vi "CodifyFrequency(Array).vi"(1 "Array":dbl[](array[numeric]) min=60.0 max=90.0 step=0.1) -> (0 "Array 2":u32[](array[numeric]))   [LabVIEW 2017, in "AODControl.lvlib"]
uses:
  AODControl.lvlib
panel:
  out "Boolean array":bool[](array[boolean])
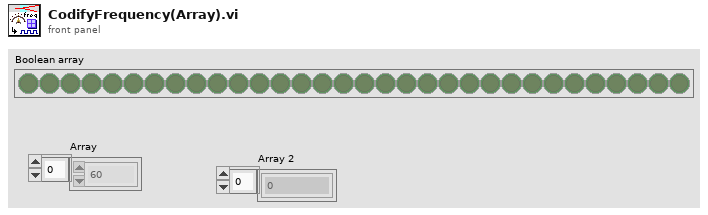
[diagram p1: front panel]
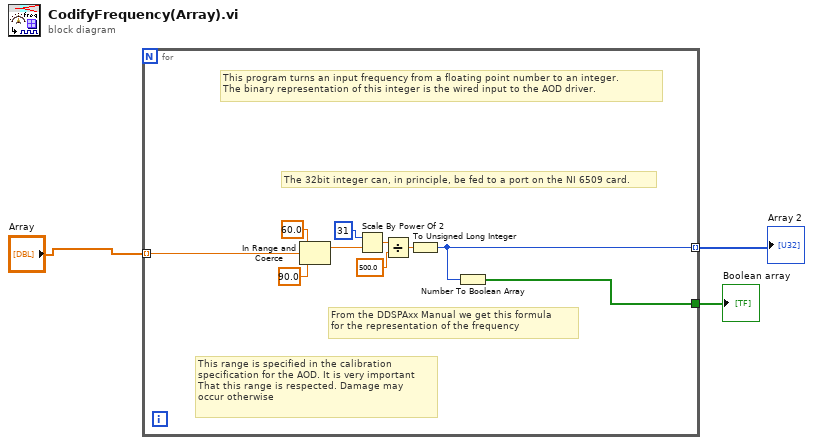
[diagram p0: block diagram]
diagram:
  n1 = for {
    tunnel: [w10] -> w3
    tunnel: "Array" -> [w8] mode=indexing
    tunnel: [w4] -> w1 mode=indexing
    # "The 32bit integer can, in principle, be fed to a port on the NI 6509 card."
    # "From the DDSPAxx Manual we get this formula\nfor the representation of the frequency"
    # "This range is specified in the calibration\nspecification for the AOD. It is very important\nThat this range is respected. Damage may \noccur otherwise"
    # "This program turns an input frequency from a floating point number to an integer. \nThe binary representation of this integer is the wired input to the AOD driver."
    n2 = In Range and Coerce(upper limit=60.0, x=w8, lower limit=90.0) -> (coerced(x)=w7:dbl)  [unwired: 1 out]
    n3 = Scale By Power Of 2(n=i16 31, x=w7) -> (x*2^n=w12:dbl)
    n4 = Divide(x=w12, y=500.0) -> (x/y=w9:dbl)
    n5 = To Unsigned Long Integer(number=w9) -> (unsigned 32bit integer=w4:u32)
    n6 = Number To Boolean Array(number=w4) -> (Boolean array=w10:bool[])
  }
  "Boolean array" <- w3
  "Array 2" <- w1
